vi "Includes Folder Auto-Populating On or Off.vi"(8 "error in":errorcluster, 10 "auto-populate (ON)":bool=TRUE, 11 "custom device path":path) -> (0 "error out":errorcluster, 3 "custom device path out":path)   [LabVIEW 2020, in "Template Tool.lvlib"]
uses:
  Template Tool.lvlib
  Template Tool Global.vi
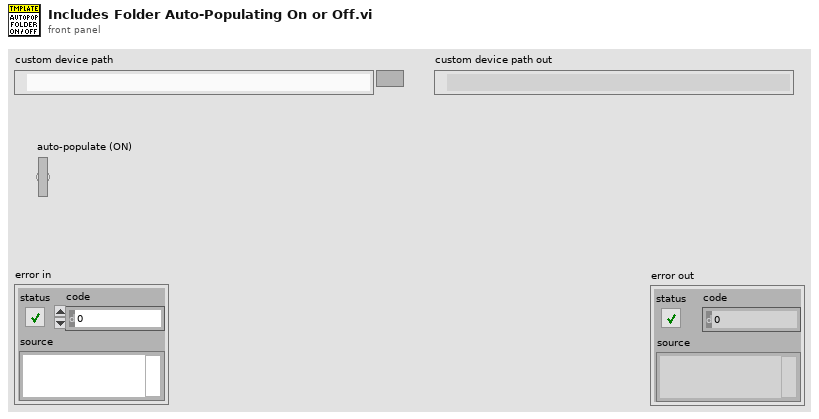
[diagram p1: front panel]
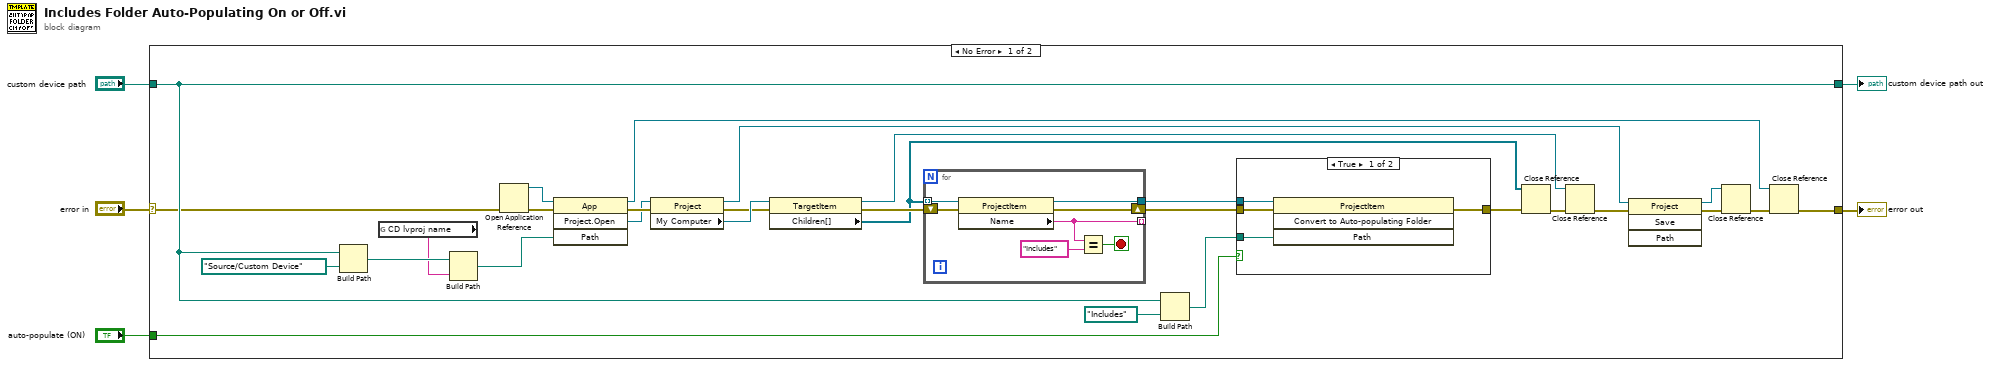
[diagram p0: block diagram]
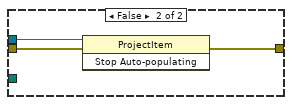
[diagram p2: hidden frame]
diagram:
  n1 = case shown="No Error" "error in" {
    selector: "error in" -> [w7 w50]
    tunnel: "custom device path" -> [w17 w49]
    tunnel: [w10 w50] -> w4
    tunnel: [w17 w49] -> w3
    tunnel: "auto-populate (ON)" -> [w15 _]
    frame No Error {
      n2 = Build Path(base path=w17, name or relative path=path "Source/Custom Device") -> (appended path=w22:path)
      n3 = global read "Template Tool Global.vi" "CD lvproj name"() -> (w8:string)
      n4 = Build Path(base path=w22, name or relative path=w8) -> (appended path=w31:path)
      n5 = Open Application Reference(8:w7) -> (0:w6:errorcluster, 3:w33:refnum<vi>)  [unwired: 3 in]
      n6 = invoke class="App" method="Project.Open"(reference=w33, error in=w6, "Path"=w31) -> (reference out=w9:refnum<vi>, error out=w23:errorcluster, "Project:Open"=w14:refnum<vi>)  [unwired: 1 in, 1 out]
      n7 = property class="Project"(reference=w14, error in=w23) -> (reference out=w13:refnum<vi>, error out=w29:errorcluster, "My Computer"=w30:refnum<vi>)
      n8 = property class="TargetItem"(reference=w30, error in=w29) -> (reference out=w28:refnum<vi>, error out=w32:errorcluster, "Children[]"=w26:refnum<vi>[])
      n9 = for {
        tunnel: w26 -> [w48] mode=indexing
        tunnel: [w47] -> _ mode=indexing
        tunnel: [w44] -> w20
        shift-right: [w42] -> w19
        shift-left: w32 -> [w43]
        stop <- w45 stop-if-true
        n10 = property class="ProjectItem"(reference=w48, error in=w43) -> (reference out=w44:refnum<vi>, error out=w42:errorcluster, "Name"=w47:string)
        n11 = Equal?(x=w47, y="Includes") -> (x = y?=w45:bool)
      }
      n12 = Build Path(base path=w17, name or relative path=path "Includes") -> (appended path=w16:path)
      n13 = case shown="True" w15 {
        tunnel: w20 -> [w38 w41]
        tunnel: w19 -> [w37 w40]
        tunnel: [w36 w39] -> w11
        tunnel: w16 -> [w35 _]
        frame True {
          n14 = invoke class="ProjectItem" method="Convert to Auto-populating Folder"(reference=w38, error in=w37, "Path"=w35) -> (error out=w36:errorcluster)  [unwired: 1 in, 3 out]
        }
        frame False {
          n15 = invoke class="ProjectItem" method="Stop Auto-populating"(reference=w41, error in=w40) -> (error out=w39:errorcluster)  [unwired: 1 in, 2 out]
        }
      }
      n16 = Close Reference(reference=w26, error in (no error)=w11) -> (error out=w27:errorcluster)
      n17 = Close Reference(reference=w28, error in (no error)=w27) -> (error out=w21:errorcluster)
      n18 = invoke class="Project" method="Save"(reference=w13, error in=w21) -> (reference out=w25:refnum<vi>, error out=w24:errorcluster)  [unwired: 2 in, 2 out]
      n19 = Close Reference(reference=w25, error in (no error)=w24) -> (error out=w12:errorcluster)
      n20 = Close Reference(reference=w9, error in (no error)=w12) -> (error out=w10:errorcluster)
    }
    frame Error {
    }
  }
  "error out" <- w4
  "custom device path out" <- w3
